vi "No1 aus Komponentenauswahl.vi"(10 "Genauigkeit":dbl, 11 "Komponentenauswahl":T1(array[cluster])) -> (3 "Komponente 1":T2 {"Komponente 5"."Komponente:" items=["NO (350,3000) LP 191C", "NO2 (150) LP 191C (1of2)", "NO2 (2000) LP 191C (2of2)", "N2O (300) LP 191C (1of2)", "NH3 (300) LP 191C (1of2)", "NH3 (900,3000) LP 191C (2of2)", "HNCO (400) 191C", "H2O% (30) LP 191C", "Formaldehyde (70,500) LP 191C", "CO2 low% (4) LP 191C (2of2)", "CO2% (20) LP 191C (1of2)", "CO (700) LP 191C (1of3)", "CO% (1) LP 191C (2of3)", "Propylene (1000) LP 191C", "Aromatic HC C7 (500) LP 191C", "Ethylene (1000) LP 191C", "CH4 (250) LP 191C (1of2)", "CH4 (5000) LP 191C (2of2)", "Ethane (1000) LP 191C", "Acetylene (1000) LP 191C", "HNO2 (20) 191C", "MeOH (1000) 191C", "CO% (10) LP 191C (3of3)", "Formic Acid (100) 191C", "SO2 (500) LP 191C", "Acetaldehyde (1000) LP 191C", "COS (100) LP 191C", "1,3 butadiene (100) LP 191C", "Oil as Octane (200) LP 191C", "N2O (1000) LP 191C (2of2)", "Propane (200) LP 191C", "NO2 autorange (2000)", "CO autorange (100000)", "CH4 autorange (5000)", "NH3 autorange (3000)", "Temp. Gascell", "Pressure Gascell", "sBeam@2500"]; "Komponente 5"."Konzentration IST" format="%#.4f"; "Komponente 5"."Genauigkeit" format="%#.1f"; "Komponente 4"."Komponente:" items=["NO (350,3000) LP 191C", "NO2 (150) LP 191C (1of2)", "NO2 (2000) LP 191C (2of2)", "N2O (300) LP 191C (1of2)", "NH3 (300) LP 191C (1of2)", "NH3 (900,3000) LP 191C (2of2)", "HNCO (400) 191C", "H2O% (30) LP 191C", "Formaldehyde (70,500) LP 191C", "CO2 low% (4) LP 191C (2of2)", "CO2% (20) LP 191C (1of2)", "CO (700) LP 191C (1of3)", "CO% (1) LP 191C (2of3)", "Propylene (1000) LP 191C", "Aromatic HC C7 (500) LP 191C", "Ethylene (1000) LP 191C", "CH4 (250) LP 191C (1of2)", "CH4 (5000) LP 191C (2of2)", "Ethane (1000) LP 191C", "Acetylene (1000) LP 191C", "HNO2 (20) 191C", "MeOH (1000) 191C", "CO% (10) LP 191C (3of3)", "Formic Acid (100) 191C", "SO2 (500) LP 191C", "Acetaldehyde (1000) LP 191C", "COS (100) LP 191C", "1,3 butadiene (100) LP 191C", "Oil as Octane (200) LP 191C", "N2O (1000) LP 191C (2of2)", "Propane (200) LP 191C", "NO2 autorange (2000)", "CO autorange (100000)", "CH4 autorange (5000)", "NH3 autorange (3000)", "Temp. Gascell", "Pressure Gascell", "sBeam@2500"]; "Komponente 4"."Konzentration IST" format="%#.4f"; "Komponente 4"."Genauigkeit" format="%#.1f"; "Komponente 3"."Komponente:" items=["NO (350,3000) LP 191C", "NO2 (150) LP 191C (1of2)", "NO2 (2000) LP 191C (2of2)", "N2O (300) LP 191C (1of2)", "NH3 (300) LP 191C (1of2)", "NH3 (900,3000) LP 191C (2of2)", "HNCO (400) 191C", "H2O% (30) LP 191C", "Formaldehyde (70,500) LP 191C", "CO2 low% (4) LP 191C (2of2)", "CO2% (20) LP 191C (1of2)", "CO (700) LP 191C (1of3)", "CO% (1) LP 191C (2of3)", "Propylene (1000) LP 191C", "Aromatic HC C7 (500) LP 191C", "Ethylene (1000) LP 191C", "CH4 (250) LP 191C (1of2)", "CH4 (5000) LP 191C (2of2)", "Ethane (1000) LP 191C", "Acetylene (1000) LP 191C", "HNO2 (20) 191C", "MeOH (1000) 191C", "CO% (10) LP 191C (3of3)", "Formic Acid (100) 191C", "SO2 (500) LP 191C", "Acetaldehyde (1000) LP 191C", "COS (100) LP 191C", "1,3 butadiene (100) LP 191C", "Oil as Octane (200) LP 191C", "N2O (1000) LP 191C (2of2)", "Propane (200) LP 191C", "NO2 autorange (2000)", "CO autorange (100000)", "CH4 autorange (5000)", "NH3 autorange (3000)", "Temp. Gascell", "Pressure Gascell", "sBeam@2500"]; "Komponente 3"."Konzentration IST" format="%#.4f"; "Komponente 3"."Genauigkeit" format="%#.1f"; "Komponente 2"."Komponente:" items=["NO (350,3000) LP 191C", "NO2 (150) LP 191C (1of2)", "NO2 (2000) LP 191C (2of2)", "N2O (300) LP 191C (1of2)", "NH3 (300) LP 191C (1of2)", "NH3 (900,3000) LP 191C (2of2)", "HNCO (400) 191C", "H2O% (30) LP 191C", "Formaldehyde (70,500) LP 191C", "CO2 low% (4) LP 191C (2of2)", "CO2% (20) LP 191C (1of2)", "CO (700) LP 191C (1of3)", "CO% (1) LP 191C (2of3)", "Propylene (1000) LP 191C", "Aromatic HC C7 (500) LP 191C", "Ethylene (1000) LP 191C", "CH4 (250) LP 191C (1of2)", "CH4 (5000) LP 191C (2of2)", "Ethane (1000) LP 191C", "Acetylene (1000) LP 191C", "HNO2 (20) 191C", "MeOH (1000) 191C", "CO% (10) LP 191C (3of3)", "Formic Acid (100) 191C", "SO2 (500) LP 191C", "Acetaldehyde (1000) LP 191C", "COS (100) LP 191C", "1,3 butadiene (100) LP 191C", "Oil as Octane (200) LP 191C", "N2O (1000) LP 191C (2of2)", "Propane (200) LP 191C", "NO2 autorange (2000)", "CO autorange (100000)", "CH4 autorange (5000)", "NH3 autorange (3000)", "Temp. Gascell", "Pressure Gascell", "sBeam@2500"]; "Komponente 2"."Konzentration IST" format="%#.4f"; "Komponente 2"."Genauigkeit" format="%#.1f"; "Komponente 1"."Komponente:" items=["NO (350,3000) LP 191C", "NO2 (150) LP 191C (1of2)", "NO2 (2000) LP 191C (2of2)", "N2O (300) LP 191C (1of2)", "NH3 (300) LP 191C (1of2)", "NH3 (900,3000) LP 191C (2of2)", "HNCO (400) 191C", "H2O% (30) LP 191C", "Formaldehyde (70,500) LP 191C", "CO2 low% (4) LP 191C (2of2)", "CO2% (20) LP 191C (1of2)", "CO (700) LP 191C (1of3)", "CO% (1) LP 191C (2of3)", "Propylene (1000) LP 191C", "Aromatic HC C7 (500) LP 191C", "Ethylene (1000) LP 191C", "CH4 (250) LP 191C (1of2)", "CH4 (5000) LP 191C (2of2)", "Ethane (1000) LP 191C", "Acetylene (1000) LP 191C", "HNO2 (20) 191C", "MeOH (1000) 191C", "CO% (10) LP 191C (3of3)", "Formic Acid (100) 191C", "SO2 (500) LP 191C", "Acetaldehyde (1000) LP 191C", "COS (100) LP 191C", "1,3 butadiene (100) LP 191C", "Oil as Octane (200) LP 191C", "N2O (1000) LP 191C (2of2)", "Propane (200) LP 191C", "NO2 autorange (2000)", "CO autorange (100000)", "CH4 autorange (5000)", "NH3 autorange (3000)", "Temp. Gascell", "Pressure Gascell", "sBeam@2500"]; "Komponente 1"."Konzentration IST" format="%#.4f"; "Komponente 1"."Genauigkeit" format="%#.1f"})   [LabVIEW 2020, in "Linearisierung v2.lvlib" / "SpanEinstellungen.lvlib"]
uses:
  SpanEinstellungen.lvlib
  Komponentencluster mit Formel.ctl
  Komponentenauswahl mit Formel.ctl
  Visualisierungs Elemente/String - Eingabefeld.ctl
  Einheit.ctl
  Gasteiler/Aktion FGV Gasteilerliste laden.ctl
  Gasteiler/Gasteiler.lvlib
panel:
  # "Komponente"
  # "Formel"
  # "Konzentration"
  # "Einheit"
  # "Genauigkeit [%]"
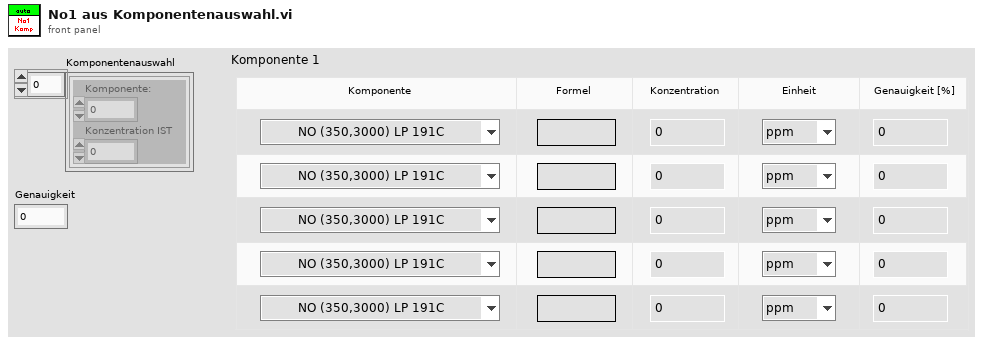
[diagram p1: front panel]
types:
  T1 = cluster{"Komponente:":u16, "Konzentration IST":dbl}[]
  T2 = typedef "Linearisierung v2.lvlib/SpanEinstellungen.lvlib/Komponentencluster mit Formel.ctl" = cluster{"Komponente 1":T3, "Komponente 2":T3, "Komponente 3":T3, "Komponente 4":T3, "Komponente 5":T3}
  T3 = typedef "Linearisierung v2.lvlib/SpanEinstellungen.lvlib/Komponentenauswahl mit Formel.ctl" = cluster{"Komponente:":u16, "Summenformel":T4, "Konzentration IST":dbl, "Einheit":T5, "Genauigkeit":dbl}
  T4 = typedef "String - Eingabefeld.ctl" = string
  T5 = typedef "Linearisierung v2.lvlib/SpanEinstellungen.lvlib/Einheit.ctl" = enum16{"ppm", "%"}
  T6 = typedef "Linearisierung v2.lvlib/Gasteiler.lvlib/Aktion FGV Gasteilerliste laden.ctl" = enum16{"lesen", "laden", "speichern", "Liste erstellen", "Formel ändern", "Gas vereinzeln"}
  T7 = cluster{"[0]":T3, "[1]":T3, "[2]":T3, "[3]":T3, "[4]":T3}
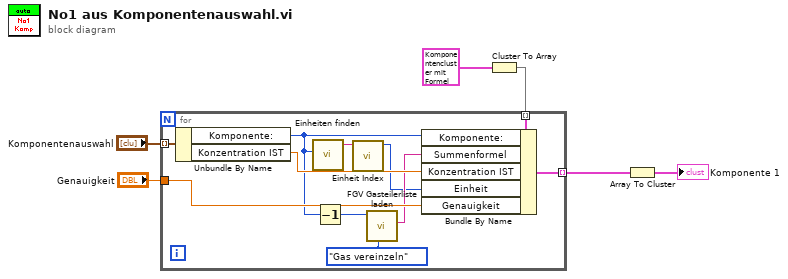
[diagram p0: block diagram]
diagram:
  n1 = Cluster To Array(cluster=T2 {"Komponente 1"={"Komponente:"=0, "Summenformel"="", "Konzentration IST"=0.0, "Einheit"=enum."ppm", "Genauigkeit"=0.0}, "Komponente 2"={"Komponente:"=0, "Summenformel"="", "Konzentration IST"=0.0, "Einheit"=enum."ppm", "Genauigkeit"=0.0}, "Komponente 3"={"Komponente:"=0, "Summenformel"="", "Konzentration IST"=0.0, "Einheit"=enum."ppm", "Genauigkeit"=0.0}, "Komponente 4"={"Komponente:"=0, "Summenformel"="", "Konzentration IST"=0.0, "Einheit"=enum."ppm", "Genauigkeit"=0.0}, "Komponente 5"={"Komponente:"=0, "Summenformel"="", "Konzentration IST"=0.0, "Einheit"=enum."ppm", "Genauigkeit"=0.0}} ("Komponente 1")) -> (array=w2:T3[])
  n2 = for {
    tunnel: "Komponentenauswahl" -> [w17] mode=indexing
    tunnel: w2 -> [w16] mode=indexing
    tunnel: [w15] -> w5 mode=indexing
    tunnel: "Genauigkeit" -> [w13]
    n3 = Unbundle By Name(w17) -> ("Komponente:"=w9:u16, "Konzentration IST"=w14:dbl)
    n4 = call "Einheiten finden.vi"("Komponente"=w9) -> ("String"=w8:string)  [unwired: 6 in, 4 out]
    n5 = Decrement(x=w9) -> (x-1=w10:u16)
    n6 = call "Einheit Index.vi"("Einheit in String"=w8) -> ("Elementindex"=w7:i32)  [unwired: 10 in]
    n7 = call "FGV Gasteilerliste laden.vi"("Aktion"=Aktion_FGV_Gasteilerliste_laden."Gas vereinzeln", "Gasindex"=w10) -> ("Formel"=w11:string)  [unwired: 7 in, 2 out]
    n8 = Bundle By Name(cluster=w16, "Komponente:"=w9, "Summenformel"=w11, "Konzentration IST"=w14, "Einheit"=w7, "Genauigkeit"=w13) -> (w15:T3)
  }
  n9 = Array To Cluster(array=w5) -> (cluster=→"Komponente 1":T7)
